vi "ProdU8.vi"(4 "Array":u8[](array[numeric])) -> (1 "Product":u8, 2 "Overflow?":bool)   [LabVIEW 2017, in "GPOverflow.lvlib"]
doc: "Multiplies all elements of <B>Array</B> keeping track of numeric overflow.\n\n<B>Overflow?</B> will be True if overflow occurred. The output will saturate in case of overflow.\n\nThis VI is inlined.\n\nSteen Schmidt\nGPower\n2/5 2014"
uses:
  GPOverflow.lvlib
panel:
  # "Copyright © 2014\nGPower\nSee enclosed license file for terms and conditions"
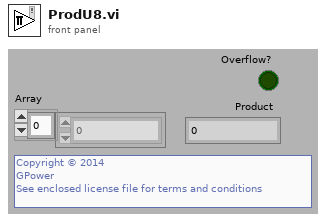
[diagram p1: front panel]
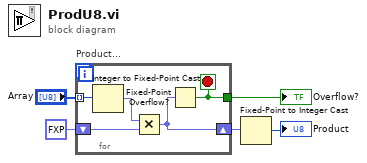
[diagram p0: block diagram]
diagram:
  n1 = for "Product..." {
    tunnel: [w8] -> w5
    tunnel: "Array" -> [w9] mode=indexing
    shift-right: [w6] -> w2
    shift-left: fxp<+,8,8> 1.0 ("fixed-point") -> [w7]
    stop <- w8 stop-if-true
    n2 = Integer to Fixed-Point Cast(integer=w9) -> (fixed-point=w10:fxp<+,8,8>)  [unwired: 1 in]
    n3 = Multiply(x=w10, y=w7) -> (x*y=w6:fxp<+,8,8>)
    n4 = Fixed-Point Overflow?(1:w6) -> (0:w8:bool)
  }
  "Overflow?" <- w5
  n5 = Fixed-Point to Integer Cast(1:w2) -> (0:→"Product":u8)
